vi "Refresh Authorization.vi"(8 "error in (no error)":errorcluster, 10 "Refresh Token":string, 11 "Oauth2 in":refnum<class "Oauth2.lvclass">) -> (0 "error out":errorcluster, 2 "Access Token":string, 3 "Oauth2 out":refnum<class "Oauth2.lvclass">)   [LabVIEW 2013, in "Oauth2.lvclass"]
uses:
  Oauth2.lvclass
  OAuthToken/OAuth2 Token Element -- enum.ctl
  Oauth2.lvclass/Oauth2.ctl
  Read RefreshToken.vi
  OAuthToken/Retrieve Element.vi
  OAuthToken/OAuthAccessToken.lvclass
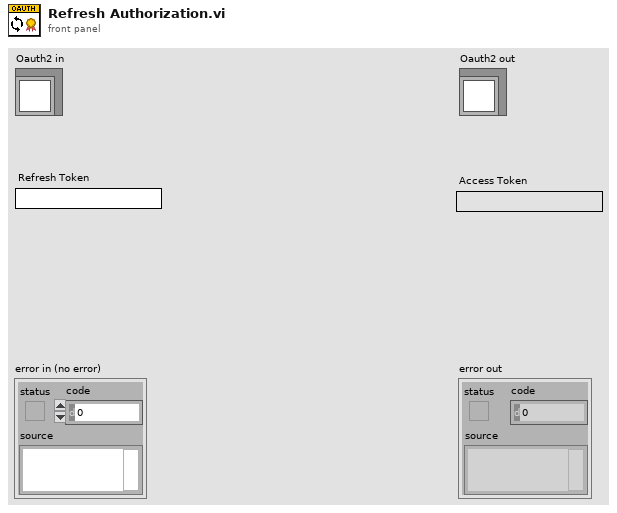
[diagram p1: front panel]
types:
  T1 = typedef "OAuthAccessToken.lvclass/OAuth2 Token Element -- enum.ctl" = enum16{"client_id", "client_secret", "response_type", "scope", "redirect_uri", "error", "error_description", "error_uri", "grant_type", "code", "access_token", "token_type", "expires_in", "username", "password", "refresh_token", "code_challenge", "code_verifier", "code_challenge_method", "endpoint element"}
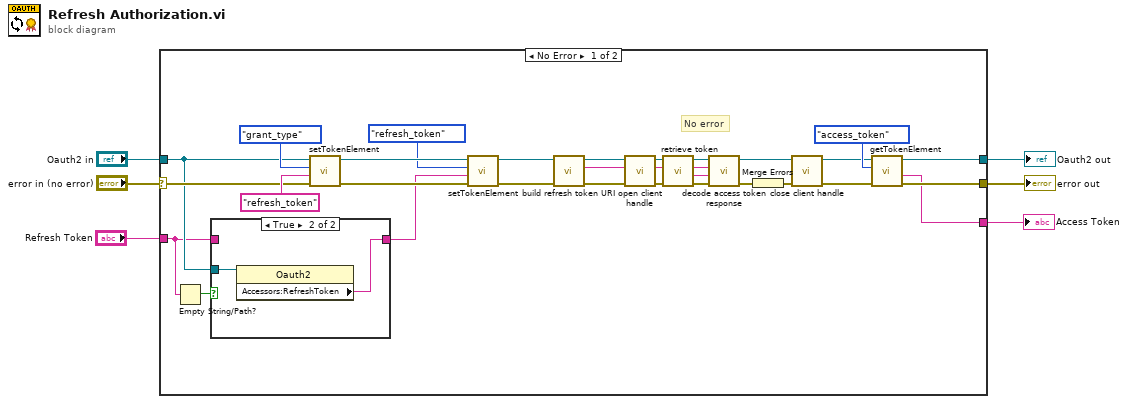
[diagram p0: block diagram]
diagram:
  n1 = case shown="No Error" "error in (no error)" {
    selector: "error in (no error)" -> [w18 w42]
    tunnel: [w36 w42] -> w5
    tunnel: [w37 w41] -> w3
    tunnel: "Oauth2 in" -> [w10 w41]
    tunnel: "Refresh Token" -> [w7 _]
    tunnel: [w33 _] -> w1
    frame No Error {
      # "No error"
      n2 = Empty String/Path?(string/path=w7) -> (empty?=w9:bool)
      n3 = case shown="True" w9 {
        tunnel: w10 -> [_ w40]
        tunnel: [w38 w39] -> w8
        tunnel: w7 -> [w38 _]
        frame False {
        }
        frame True {
          n4 = property class="Oauth2"(reference=w40) -> ("Accessors:RefreshToken"=w39:string)  [unwired: 1 in, 2 out]
        }
      }
      n5 = call "setTokenElement.vi"("error in (no error)"=w18, "Value"="refresh_token", "Token element"=OAuth2_Token_Element_--_enum."grant_type", "Oauth2 in"=w10) -> ("error out"=w19:errorcluster, "Oauth2 out"=w17:refnum<class "Oauth2.lvclass">)  [unwired: 6 in]
      n6 = call "setTokenElement.vi"("error in (no error)"=w19, "Value"=w8, "Token element"=OAuth2_Token_Element_--_enum."refresh_token", "Oauth2 in"=w17) -> ("error out"=w14:errorcluster, "Oauth2 out"=w15:refnum<class "Oauth2.lvclass">)  [unwired: 6 in]
      n7 = call-dynamic "build refresh token URI.vi"("error in (no error)"=w14, "Oauth2 in"=w15) -> ("error out"=w11:errorcluster, "Refresh Token Request URI"=w13:string, "Oauth2"=w12:refnum<class "Oauth2.lvclass">)  [unwired: 7 in]
      n8 = call "open client handle.vi"("error in (no error)"=w11, "Request URI in"=w13, "Oauth2 in"=w12) -> ("error out"=w30:errorcluster, "Request URI dup"=w29:string, "Oauth2 out"=w31:refnum<class "Oauth2.lvclass">)  [unwired: 6 in]
      n9 = call "retrieve token.vi"("error in (no error)"=w30, "Token Request URI"=w29, "Oauth2 in"=w31) -> ("error out"=w26:errorcluster, "Response"=w23:string, "Header"=w24:string, "Oauth2 out"=w28:refnum<class "Oauth2.lvclass">)  [unwired: 5 in]
      n10 = call-dynamic "decode access token response.vi"("error in (no error)"=w26, "Response"=w23, "Header"=w24, "Oauth2 in"=w28) -> ("error out"=w25:errorcluster, "Oauth2"=w27:refnum<class "Oauth2.lvclass">)  [unwired: 6 in]
      n11 = Merge Errors(w25) -> (w32:errorcluster)
      n12 = call "close client handle.vi"("error in (no error)"=w32, "Oauth2 in"=w27) -> ("error out"=w22:errorcluster, "Oauth2 out"=w34:refnum<class "Oauth2.lvclass">)  [unwired: 8 in]
      n13 = call "getTokenElement.vi"("error in (no error)"=w22, "Token element"=OAuth2_Token_Element_--_enum."access_token", "Oauth2 in"=w34) -> ("error out"=w36:errorcluster, "Value"=w33:string, "Oauth2 out"=w37:refnum<class "Oauth2.lvclass">)  [unwired: 5 in, 1 out]
    }
    frame Error {
    }
  }
  "error out" <- w5
  "Oauth2 out" <- w3
  "Access Token" <- w1
